vi "Agilent 34401 Acquire and Chart - Pretriggered.vi"() -> ()   [LabVIEW 2015]
doc: "This example shows how to configure a pretriggered measurement using the low-level Data VIs to retrieve data from the DMM. Measurements are obtained from the instrument's internal buffer and are read iteratively and charted.\n\n<B>Note:</B>\n\n(1) This VI only applies to the Agilent 34411 model.\n\n(2) It is recommended that all triggered measurements be made using an appropriate fixed manual range. That is, disable autorange and manually select a range in <B>Configure Measurement VI</B>."
uses:
  <vilib>/Utility/error.llb/DialogType.ctl
  <instrlib>/Agilent 34401/Agilent 34401.lvlib
panel:
  in  "Slope (0: Negative)":u16(ring) items=["Negative", "Positive"]
  in  "Trigger Source (0: Immediate)":u16(ring) items=["Immediate", "Software (Bus)", "External", "Internal"]
  in  "Function (0: DC Voltage)":u16(ring) items=["DC Voltage", "AC Voltage", "2 - Wire Resistance", "4 - Wire Resistance", "DC Current", "AC Current", "Frequency", "Period", "Continuity", "Diode Checking", "VDC:VDC Ratio", "Temperature", "Capacitance"]
  out "Measurements":dbl[](graph)
  in  "Stop":bool
  in  "Internal Level (0)":dbl
  in  "VISA resource name":refnum<visa-resource-name>
  in  "Sample Count (20)":i32=20 format="%#.6g"
  in  "Pretrigger Samples (10)":i32=10
  in  "Manual Range (1.00)":dbl=1.0 format="%_3f"
  # "(c) 2005-2015 National Instruments.  ALL RIGHTS RESERVED."
  # "Note: This VI only applies to the 34411A model"
  # "Note: Sample Count must be greater than Pretrigger Samples."
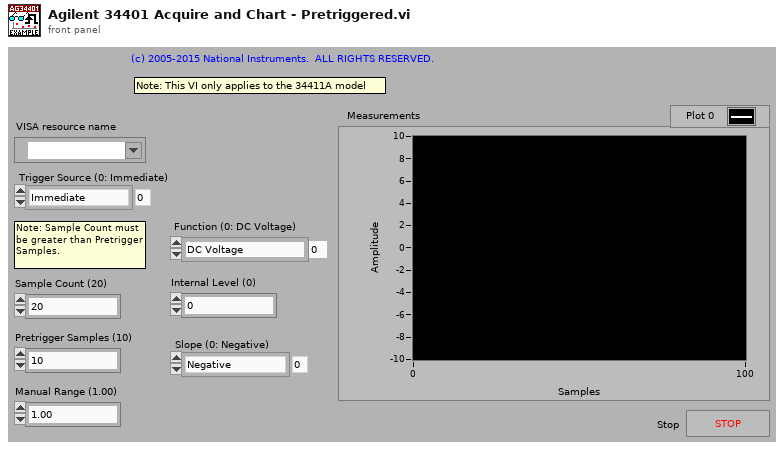
[diagram p1: front panel]
types:
  T1 = typedef "DialogType.ctl" = u16
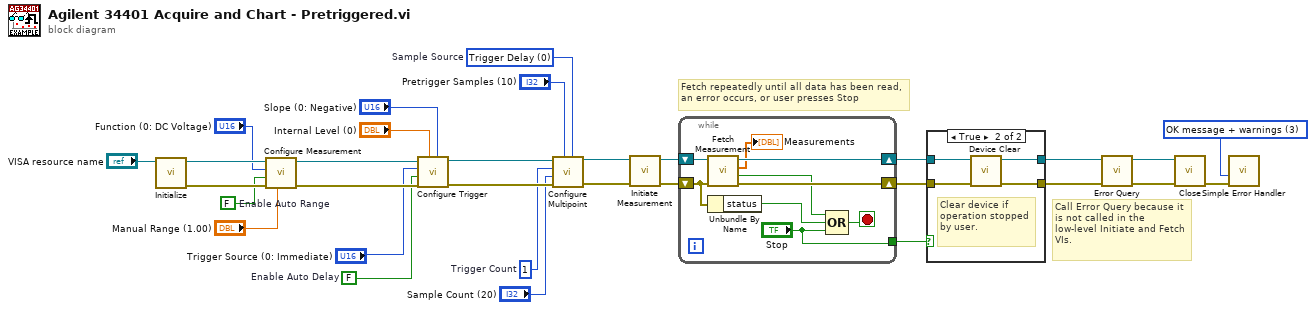
[diagram p0: block diagram]
diagram:
  w11 = T1 3 items=["no dialog", "OK message", "continue or stop message", "OK message + warnings", "continue/stop + warnings"] ("type of dialog (OK msg:1)")
  w18 = 1  # Trigger Count
  w19 = u16 0 items=["Trigger Delay", "Sample Interval"]  # Sample Source
  w23 = FALSE  # Enable Auto Delay
  w25 = FALSE  # Enable Auto Range
  # "Call Error Query because it is not called in the low-level Initiate and Fetch VIs."
  # "Fetch repeatedly until all data has been read, an error occurs, or user presses Stop"
  n1 = call <instrlib>:"Initialize.vi"("VISA resource name"="VISA resource name") -> ("error out"=w31:errorcluster, "VISA resource name out"=w30:refnum<visa-resource-name>)  [unwired: 9 in]
  n2 = call <instrlib>:"Configure Measurement.vi"("Manual Range (1.00)"="Manual Range (1.00)", "error in (no error)"=w31, "Enable Auto Range (T: Enable)"=w25, "Function (0: DC Voltage)"="Function (0: DC Voltage)", "VISA resource name"=w30) -> ("error out"=w29:errorcluster, "VISA resource name out"=w28:refnum<visa-resource-name>)  [unwired: 5 in]
  n3 = call <instrlib>:"Configure Trigger.vi"("Slope (0: Negative)"="Slope (0: Negative)", "Internal Level (0)"="Internal Level (0)", "error in (no error)"=w29, "Enable Auto Delay (T: Enable)"=w23, "Trigger Source (0: Immediate)"="Trigger Source (0: Immediate)", "VISA resource name"=w28) -> ("error out"=w27:errorcluster, "VISA resource name out"=w26:refnum<visa-resource-name>)  [unwired: 4 in]
  n4 = call <instrlib>:"Configure Multipoint.vi"("Sample Source (0:Trigger Delay)"=w19, "Pretrigger Samples (0)"="Pretrigger Samples (10)", "error in (no error)"=w27, "Sample Count (1)"="Sample Count (20)", "Trigger Count (1)"=w18, "VISA resource name"=w26) -> ("error out"=w21:errorcluster, "VISA resource name out"=w20:refnum<visa-resource-name>)  [unwired: 4 in]
  n5 = call <instrlib>:"Initiate Measurement.vi"("error in (no error)"=w21, "VISA resource name"=w20) -> ("error out"=w12:errorcluster, "VISA resource name out"=w13:refnum<visa-resource-name>)  [unwired: 8 in]
  n6 = while {
    tunnel: ["Stop"] -> w8
    shift-right: [w40] -> w9
    shift-left: w13 -> [w38]
    shift-right: [w39] -> w10
    shift-left: w12 -> [w34]
    stop <- w36 stop-if-true
    n7 = call <instrlib>:"Fetch Measurement.vi"("error in (no error)"=w34, "VISA resource name"=w38) -> ("error out"=w39:errorcluster, "End of Data?"=w37:bool, "Measurements"=→"Measurements":dbl[], "VISA resource name out"=w40:refnum<visa-resource-name>)  [unwired: 6 in]
    n8 = Unbundle By Name(w34) -> ("status"=w33:bool)
    n9 = Compound Arithmetic op=OR(w37, w33, "Stop") -> (w36:bool)
  }
  n10 = case shown="True" w8 {
    tunnel: w9 -> [w42 w46]
    tunnel: w10 -> [w41 w45]
    tunnel: [w42 w44] -> w5
    tunnel: [w41 w43] -> w4
    frame False {
    }
    frame True {
      # "Clear device if operation stopped by user."
      n11 = call <instrlib>:"Device Clear.vi"("error in (no error)"=w45, "VISA Resource Name"=w46) -> ("error out"=w43:errorcluster, "VISA Resource Out"=w44:refnum<visa-resource-name>)  [unwired: 8 in]
    }
  }
  n12 = call <instrlib>:"Error Query.vi"("error in (no error)"=w4, "VISA resource name"=w5) -> ("error out"=w7:errorcluster, "VISA resource name out"=w6:refnum<visa-resource-name>)  [unwired: 6 in, 2 out]
  n13 = call <instrlib>:"Close.vi"("error in (no error)"=w7, "VISA resource name"=w6) -> ("error out"=w14:errorcluster)  [unwired: 9 in]
  n14 = call <vilib>:"Simple Error Handler.vi"("type of dialog (OK msg:1)"=w11, "error in (no error)"=w14) -> ()  [unwired: 3 in, 5 out]
